vi "Get dstp Reply Loaction.vi"(8 "error in":errorcluster, 11 "Reply Protocol DataSocket in":refnum<class "Reply Protocol DataSocket.lvclass">) -> (0 "error out":errorcluster, 2 "Reply Location":string, 3 "Reply Protocol DataSocket out":refnum<class "Reply Protocol DataSocket.lvclass">)   [LabVIEW 2023, in "HAL GOOP4.lvlib" / "Reply Protocol DataSocket.lvclass"]
uses:
  Reply Protocol DataSocket.lvclass
  Reply Protocol DataSocket.lvclass/Reply Protocol DataSocket.ctl
  Reply Protocol Base/Reply Protocol Base.lvclass/Reply Protocol Base.ctl
  Reply Protocol Base/Reply Protocol Base.lvclass
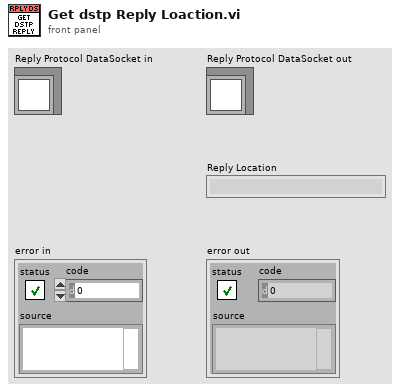
[diagram p1: front panel]
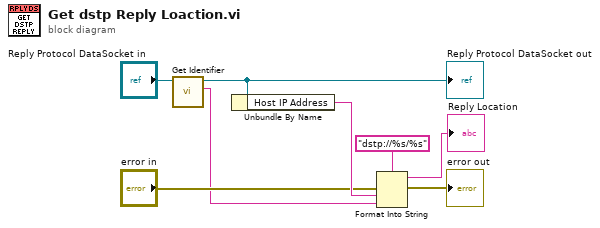
[diagram p0: block diagram]
diagram:
  n1 = call "Get Identifier.vi"("Reply Protocol Base in"="Reply Protocol DataSocket in") -> ("Identifier"=w1:string, "Reply Protocol Base out"=w4:refnum<class "Reply Protocol DataSocket.lvclass">)  [unwired: 9 in]
  "Reply Protocol DataSocket out" <- w4
  n2 = Unbundle By Name(w4) -> ("Host IP Address"=w8:string)
  n3 = Format Into String(format string="dstp://%s/%s", error in="error in", w8, w1) -> (resulting string=→"Reply Location":string, error out=→"error out":errorcluster)  [unwired: 1 in]
